vi "v0.2_RPM_acelerar_serial.vi"(4 "PA:13":u32=1, 6 "PA:12":u32=1, 7 "tiempo_ms":i32, 8 "error_in":errorcluster, 9 "RPM_Inicio":u32, 10 "RPM_Final":u32, 11 "VISA COM IN":refnum<visa-resource-name>) -> (0 "error out":errorcluster, 2 "FQ_salida":u32, 3 "VISA COM OUT":refnum<visa-resource-name>)   [LabVIEW 2011]
doc: "<B>Acelerar mediante PTO</B>\n\nEste VI se utiliza para acelerar la <B>frecuencia</B> del tren de pulsos. Envia un nuevo comando cada 1ms hasta alcanzar la frecuencia deseada."
uses:
  <vilib>/Platform/TimedLoop/XDataNode/timing_clust.ctl
  <vilib>/Platform/TimedLoop/XDataNode/nitl_modes.ctl
  <vilib>/Platform/TimedLoop/XDataNode/wakeup.ctl
  <vilib>/Platform/TimedLoop/XDataNode/XDataNode.xnode
  <vilib>/Platform/TimedLoop/XDataNode/XDNodeRunTimeDep.lvlib
panel:
  # "FUNCION ACELERACIÓN PARA LA FRECUENCIA DE SALIDA"
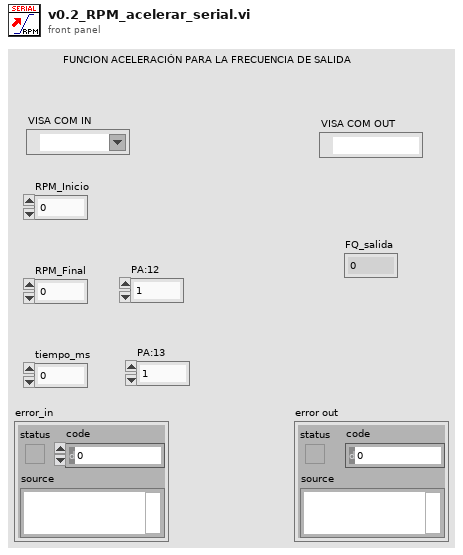
[diagram p1: front panel]
types:
  T1 = typedef "XDNodeRunTimeDep.lvlib/timing_clust.ctl" = cluster{"Expected End [f-1]":u64, "Actual End [f-1]":u64, "Finished Late? [f-1]":bool, "Expected End [i-1]":u64, "Actual End [i-1]":u64, "Finished Late? [i-1]":bool, "Expected Start [i]":u64, "Actual Start [i]":u64, "Expected Start [f]":u64, "Actual Start [f]":u64, "Source Name":string, "Structure Name":string, "Period":i64, "Deadline":i64, "Offset":i64, "Start":i64, "Priority":i32, "Timeout":i32, "Mode":T2, "Wakeup Reason":T3, "Error":errorcluster, "Source Type":string, "Secondary Source Type":string, "Global End Time":u64, "Global Start Time":u64, "Frame Duration":u64, "Iteration Duration":u64, "Assigned CPU":i32, "I/O Scan Engine Mode":u32}
  T2 = typedef "XDNodeRunTimeDep.lvlib/nitl_modes.ctl" = enum32{"No Change", "Process missed periods, maintain original phase", "Discard missed periods, maintain original phase", "Process missed periods, ignore original phase", "Discard missed periods, ignore original phase"}
  T3 = typedef "XDNodeRunTimeDep.lvlib/wakeup.ctl" = enum32{"Normal", "Aborted", "Asynchronous wakeup", "Timing source error", "Timed loop error", "Timeout"}
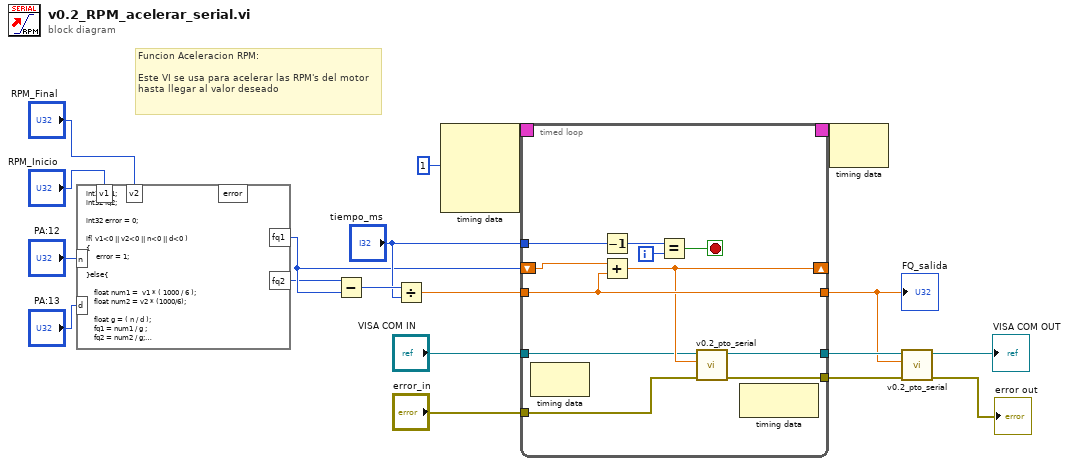
[diagram p0: block diagram]
diagram:
  # "Funcion Aceleracion RPM:\n\nEste VI se usa para acelerar las RPM's del motor\nhasta llegar al valor deseado"
  n1 = formula code="int32 fq1;\nint32 fq2;\n\nint32 error = 0;\n\nif( v1<0 || v2<0 || n<0 || d<0 )\n{\n     error = 1; \n\n}else{\n\n    float num1 =  v1 * ( 1000 / 6 );\n    float num2 = v2 * (1000/6);\n\n    float g = ( n / d );\n    fq1 = num1 / g ;\n    fq2 = num2 / g;\n}"("v1"="RPM_Inicio", "n"="PA:12", "d"="PA:13", "v2"="RPM_Final") -> ("fq1"=w3:i32, "fq2"=w1:i32)  [unwired: 1 out]
  n2 = Subtract(x=w1, y=w3) -> (x-y=w19:i32)
  n3 = Divide(x=w19, y="tiempo_ms") -> (x/y=w14:dbl)
  n4 = node-c288(i64 1 ("Period")) -> (w18:T1)  [unwired: 3 in]
  n5 = timed-loop {
    timing: w18 -> [_]
    timing-out: [_] -> w17
    tunnel: "tiempo_ms" -> [w28]
    shift-right: [w24] -> _
    shift-left: w3 -> [w26]
    tunnel: w14 -> [w25]
    tunnel: "VISA COM IN" -> [w23]
    tunnel: [w22] -> w12
    tunnel: [w25] -> w10
    tunnel: [w20] -> w11
    tunnel: "error_in" -> [w21]
    i -> [w30]
    stop <- w29 stop-if-true
    n6 = node-c288() -> ()  [unwired: 1 in, 1 out]
    n7 = Decrement(x=w28) -> (x-1=w27:i32)
    n8 = Add(x=w26, y=w25) -> (x+y=w24:dbl)
    n9 = Equal?(x=w27, y=w30) -> (x = y?=w29:bool)
    n10 = call "v0.2_pto_serial.vi"("error in (no error)"=w21, "Fout"=w24, "VISA COM IN"=w23) -> ("error out"=w20:errorcluster, "VISA COM OUT"=w22:refnum<visa-resource-name>)  [unwired: 7 in]
    n11 = node-c288() -> ()  [unwired: 1 in, 1 out]
  }
  "FQ_salida" <- w10
  n12 = node-c288(w17) -> ()  [unwired: 1 out]
  n13 = call "v0.2_pto_serial.vi"("error in (no error)"=w11, "Fout"=w10, "VISA COM IN"=w12) -> ("error out"=→"error out":errorcluster, "VISA COM OUT"=→"VISA COM OUT":refnum<visa-resource-name>)  [unwired: 7 in]
